vi "断电保存全局.vi"() -> ()   [LabVIEW 2016, in "质控单元.lvlib"]
uses:
  <vilib>/Plasmionique/MB Master/MB_Master_TCP/MB_Master_TCP.lvclass
  <vilib>/Plasmionique/MB Master/MB_Master/MB_Master.lvclass
panel:
  in  "Slave ID":T1={"氨氮"=1, "总磷"=2, "总氮"=3, "CODMn"=4, "CODCr"=5}
  in  "模块组合":enum16{"氨氮总磷", "总磷总氮", "氨氮、总磷、总氮"}(ring)=enum."氨氮、总磷、总氮"
  in  "定时控制":T2
  out "MB session out":refnum<class "MB_Master.lvclass">
  out "MB_TCP session":refnum<class "MB_Master_TCP.lvclass">
  in  "PORT":string="1005"
  in  "IP":string="127.0.0.1"
  in  "MB通信方式选择":enum16{"串口", "TCP"}(ring)
  in  "Serial Config":T3={"baud rate (bps)"=115200, "stop bits"=10, "parity"=0, "flow control"=0, "timeout"=100, "retries"=1} {"stop bits" items=["1.0"=10, "1.5"=15, "2.0"=20]; "parity" items=["None", "Odd", "Even", "Mark", "Space"]; "flow control" items=["None", "XON/XOFF", "RTS/CTS", "XON/XOFF & RTS/CTS", "DTR/DSR", "XON/XOFF & DTR/DSR"]}
  in  "VISA Resource":refnum<visa-resource-name>="COM8"
  in  "CODCr选择":bool
  in  "CODMn选择":bool
  in  "总磷总氮模块选择":bool
  in  "氨氮模块":bool
  in  "CODCr量程选择":enum32{"H", "L", "AUTO"}(ring)
  in  "CODMn量程选择":enum32{"H", "L", "AUTO"}(ring)
  in  "总磷量程选择":enum32{"H", "L", "AUTO"}(ring)=enum."AUTO"
  in  "总氮量程选择":enum32{"H", "L", "AUTO"}(ring)=enum."AUTO"
  in  "氨氮量程选择":enum32{"H", "L", "AUTO"}(ring)=enum."AUTO"
  # "MBTCP参数"
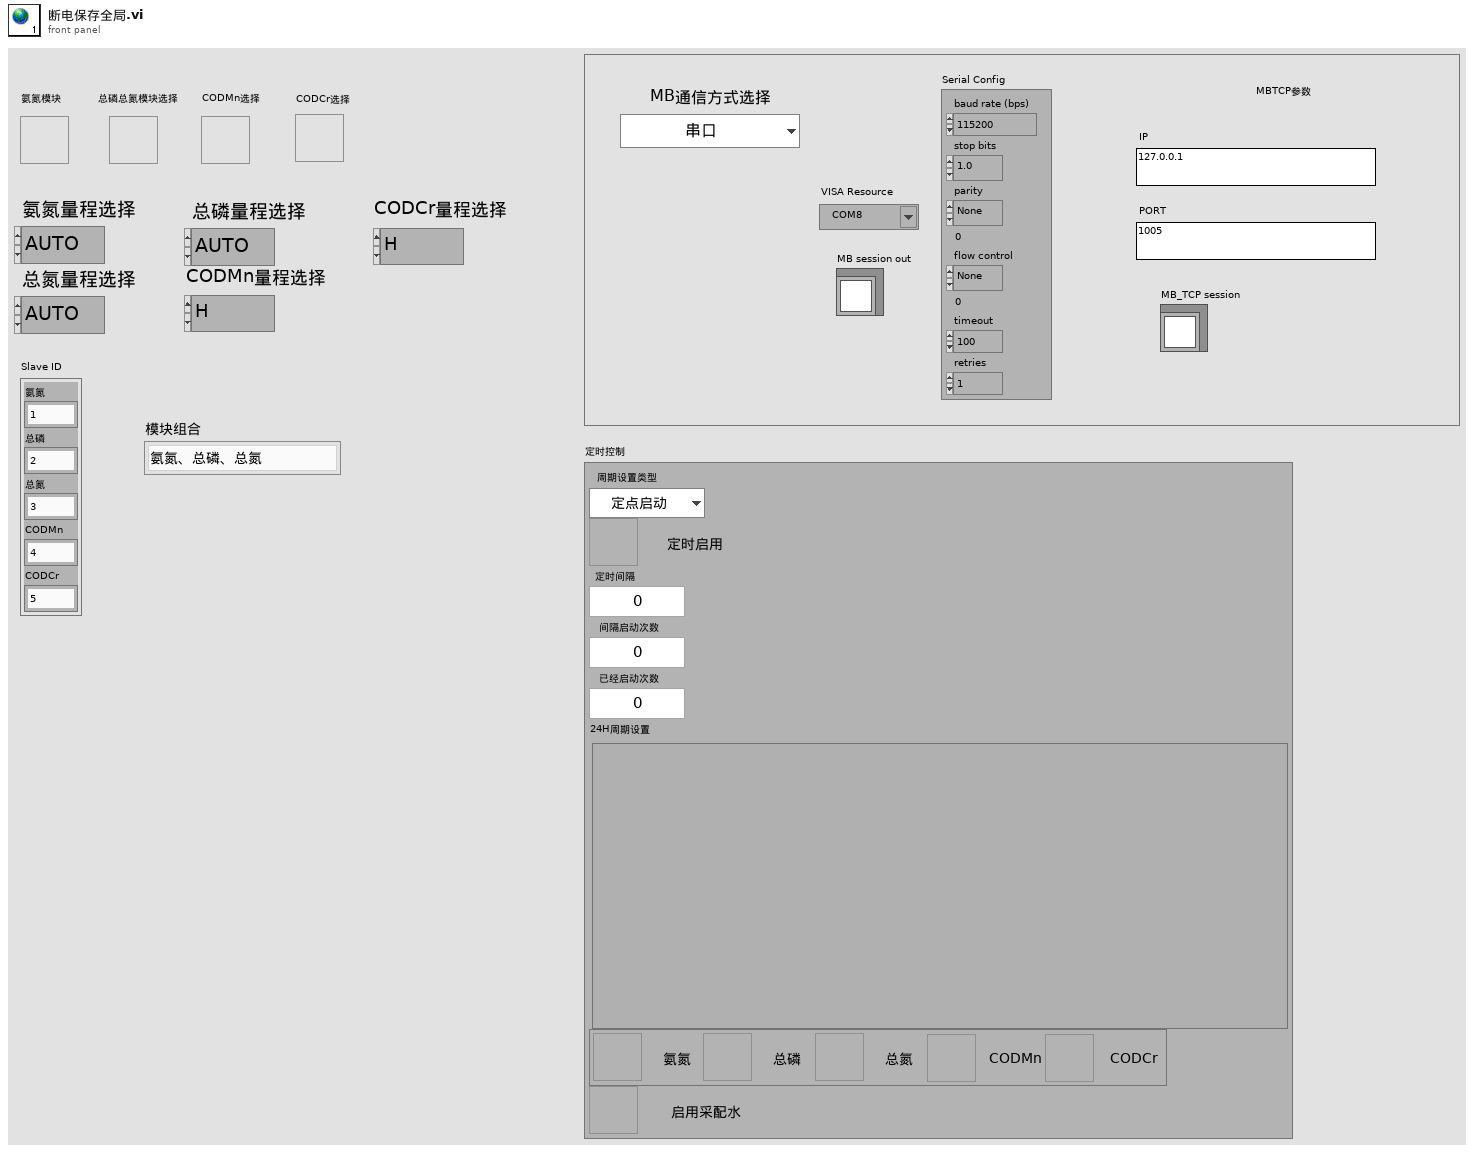
[diagram p1: front panel]
types:
  T1 = cluster{"氨氮":u8, "总磷":u8, "总氮":u8, "CODMn":u8, "CODCr":u8}
  T2 = cluster{"周期设置类型":enum16{"定点启动", "间隔启动"}, "定时功能启用":bool, "定时间隔":dbl, "间隔启动次数 ":dbl, "已经启动次数 ":dbl, "24H周期设置":bool[], "模块选择":cluster{"氨氮":bool, "总磷":bool, "总氮":bool, "CODMn":bool, "CODCr":bool}, "采配水启用":bool}
  T3 = cluster{"baud rate (bps)":u32, "stop bits":u16, "parity":u16, "flow control":u16, "timeout":u32, "retries":i32}
diagram:
